vi "ADC 3ch Example LaunchPad.vi"() -> ()   [LabVIEW 2011]
panel:
  in  "stop":bool
  in  "Update Interval (ms)":u32(knob)=1009 scale=150.0..5000.0
  out "Z Chart":dbl(graph)
  out "Y Chart":dbl(graph)
  out "X Chart":dbl(graph)
  out "CurrentPath":path=path "C:/Documents and Settings/TGI0362/My Documents/xUserData/LabVIEW_8.x/cmDVT_Factory-BBU-R5"
  out "new picture":picture
  # "3 channel ADC example\nwtih adjustable sampling time delay"
  # "X"
  # "Y"
  # "Z"
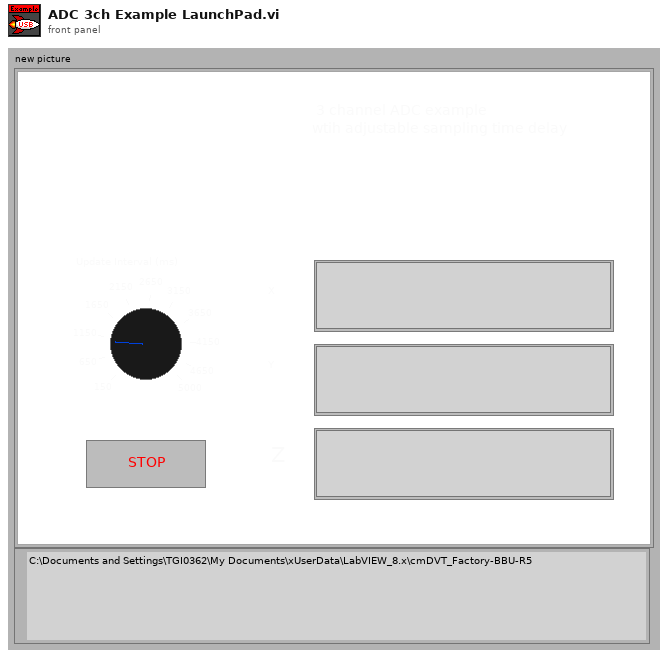
[diagram p1: front panel]
types:
  T1 = typedef "imagedata.ctl" = cluster{"image type":i32, "image depth":i32, "image":u8[], "mask":u8[], "colors":u32[], "Rectangle":cluster{"left":i16, "top":i16, "right":i16, "bottom":i16}}
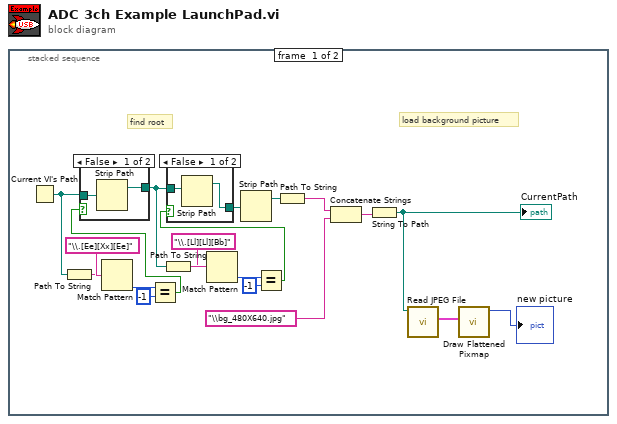
[diagram p0: block diagram]
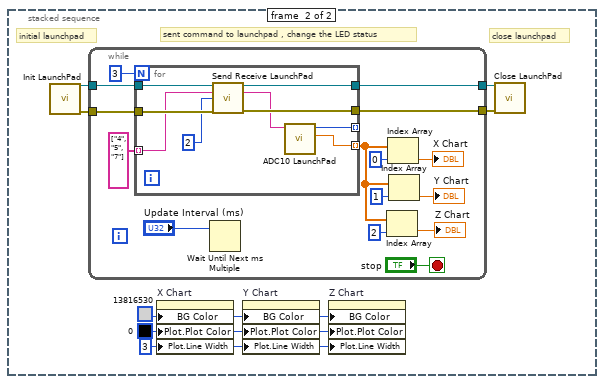
[diagram p4: hidden frame]
diagram:
  n1 = stacked-sequence {
    frame #0 {
      # "load background picture"
      # "find root"
      n2 = Current VI's Path() -> (path=w9:path)
      n3 = Path To String(path=w9) -> (string=w8:string)
      n4 = Match Pattern(string=w8, regular expression="\\.[Ee][Xx][Ee]") -> (offset past match=w6:i32)  [unwired: 1 in, 3 out]
      n5 = Equal?(x=w6, y=-1) -> (x = y?=w18:bool)
      n6 = case shown="False" w18 {
        tunnel: [w24 w26] -> w15
        tunnel: w9 -> [w25 w26]
        frame False {
          n7 = Strip Path(path=w25) -> (stripped path=w24:path)  [unwired: 1 out]
        }
        frame True {
        }
      }
      n8 = Path To String(path=w15) -> (string=w12:string)
      n9 = Match Pattern(string=w12, regular expression="\\.[Ll][Ll][Bb]") -> (offset past match=w14:i32)  [unwired: 1 in, 3 out]
      n10 = Equal?(x=w14, y=-1) -> (x = y?=w17:bool)
      n11 = case shown="False" w17 {
        tunnel: [w21 w23] -> w16
        tunnel: w15 -> [w22 w23]
        frame False {
          n12 = Strip Path(path=w22) -> (stripped path=w21:path)  [unwired: 1 out]
        }
        frame True {
        }
      }
      n13 = Strip Path(path=w16) -> (stripped path=w5:path)  [unwired: 1 out]
      n14 = Path To String(path=w5) -> (string=w2:string)
      n15 = Concatenate Strings(w2, "\\bg_480X640.jpg") -> (w3:string)
      n16 = String To Path(string=w3) -> (path=w1:path)
      "CurrentPath" <- w1
      n17 = call <vilib>:"Read JPEG File.vi"("path to JPEG file"=w1) -> ("image data"=w19:T1)  [unwired: 8 in, 2 out]
      n18 = call <vilib>:"Draw Flattened Pixmap.vi"("image data"=w19) -> ("new picture"=→"new picture":picture)  [unwired: 8 in]
    }
    frame #1 {
      w27 = 3
      w28 = u32 0
      w29 = u32 13816530
      # "close launchpad"
      # "sent command to launchpad , change the LED status"
      # "initial launchpad"
      n19 = call "Init LaunchPad.vi"() -> ("error out"=w32:errorcluster, "VISA resource name out"=w33:refnum<visa-resource-name>)  [unwired: 10 in]
      n20 = while {
        tunnel: w33 -> [w48]
        tunnel: w32 -> [w47]
        tunnel: [w44] -> w31
        tunnel: [w43] -> w30
        stop <- "stop" stop-if-true
        n21 = for {
          N: 3 -> [_]
          tunnel: w48 -> [w57]
          tunnel: [w56] -> w44
          tunnel: [w55] -> w43
          tunnel: w47 -> [w54]
          tunnel: string[] ["4", "5", "7"] -> [w52] mode=indexing
          tunnel: [w50] -> _ mode=indexing
          tunnel: [w49] -> w38 mode=indexing
          n22 = call "Send Receive LaunchPad.vi"("VISA resource"=w57, "write buffer"=w52, "Bytes To Read (0)"=u8 2, "error in"=w54) -> ("VISA resource 2"=w56:refnum<visa-resource-name>, "Read Buffer"=w51:string, "error out"=w55:errorcluster)  [unwired: 9 in]
          n23 = call "ADC10 LaunchPad.vi"("string"=w51) -> ("ADC10 (Volt)"=w49:dbl, "ADCvalue"=w50:u16)  [unwired: 9 in]
        }
        n24 = Wait Until Next ms Multiple(millisecond multiple="Update Interval (ms)") -> ()  [unwired: 1 out]
        n25 = Index Array(array=w38, index=2) -> (element=→"Z Chart":dbl)
        n26 = Index Array(array=w38, index=0) -> (element=→"X Chart":dbl)
        n27 = Index Array(array=w38, index=1) -> (element=→"Y Chart":dbl)
      }
      n28 = property on="X Chart" class="WFChart (strict)"("BG Color"=w29, "Plot.Plot Color"=w28, "Plot.Line Width"=w27) -> ()  [unwired: 2 in, 2 out]
      n29 = property on="Y Chart" class="WFChart (strict)"("BG Color"=w29, "Plot.Plot Color"=w28, "Plot.Line Width"=w27) -> ()  [unwired: 2 in, 2 out]
      n30 = property on="Z Chart" class="WFChart (strict)"("BG Color"=w29, "Plot.Plot Color"=w28, "Plot.Line Width"=w27) -> ()  [unwired: 2 in, 2 out]
      n31 = call "Close LaunchPad.vi"("VISA resource name"=w31, "error in"=w30) -> ()  [unwired: 13 in, 1 out]
    }
  }
